vi "cont_array_float.vi"(7 "ignore_first_edge?":bool, 8 "edge cluster":cluster{"Array":i16[], "Array":bool[]}, 11 "u8_ar_phase map":dbl[](array[numeric])) -> (3 "Array":dbl[](array[numeric]))   [LabVIEW 2011]
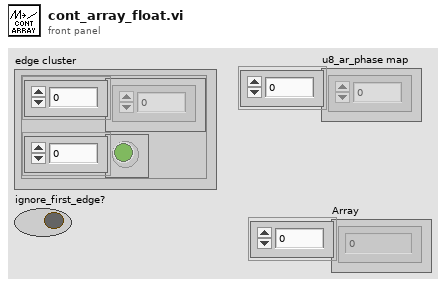
[diagram p1: front panel]
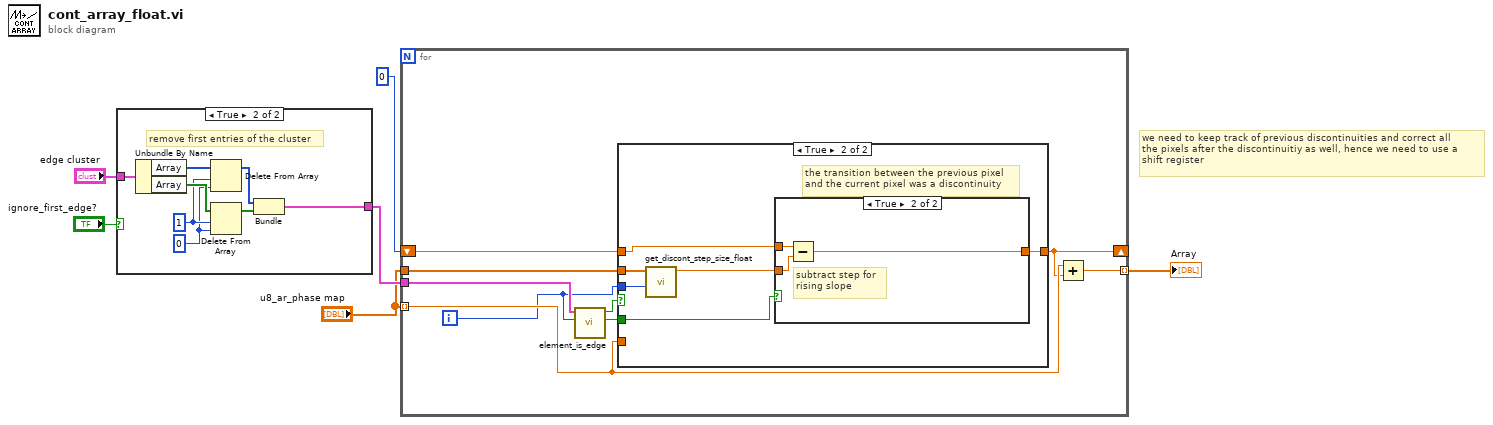
[diagram p0: block diagram]
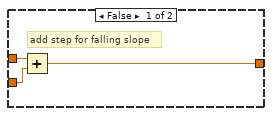
[diagram p4: hidden frame]
diagram:
  # "we need to keep track of previous discontinuities and correct all \nthe pixels after the discontinuitiy as well, hence we need to use a \nshift register"
  n1 = case shown="True" "ignore_first_edge?" {
    tunnel: "edge cluster" -> [w7 w9]
    tunnel: [w7 w8] -> w3
    frame False {
    }
    frame True {
      w13 = 1 ("length")
      w12 = 0 ("index")
      # "remove first entries of the cluster"
      n2 = Unbundle By Name(w9) -> ("Array"=w15:i16[], "Array"=w14:bool[])
      n3 = Delete From Array(array=w15, length=w13, index=w12) -> (array with subset deleted=w11:i16[])  [unwired: 1 out]
      n4 = Delete From Array(array=w14, length=w13, index=w12) -> (array with subset deleted=w10:bool[])  [unwired: 1 out]
      n5 = Bundle("Array"=w11, "Array"=w10) -> (w8:cluster{"Array":i16[], "Array":bool[]})  [unwired: 1 in]
    }
  }
  n6 = for {
    tunnel: "u8_ar_phase map" -> [w20]
    tunnel: "u8_ar_phase map" -> [w22] mode=indexing
    shift-right: [w19] -> _
    shift-left: i16 0 -> [w24]
    tunnel: [w23] -> w5 mode=indexing
    tunnel: w3 -> [w21]
    i -> [w18]
    n7 = call "element_is_edge.vi"("current element"=w18, "edge cluster"=w21) -> ("direction (rising/falling)"=w16:bool, "edge"=w17:bool)  [unwired: 8 in]
    n8 = case shown="True" w17 {
      tunnel: [w25 w30] -> w19
      tunnel: w24 -> [w25 w31]
      tunnel: w16 -> [_ w29]
      tunnel: w22 -> [_ _]
      tunnel: w18 -> [_ w27]
      tunnel: w20 -> [_ w28]
      frame False {
      }
      frame True {
        # "the transition between the previous pixel\nand the current pixel was a discontinuity"
        n9 = call "get_discont_step_size_float.vi"("current pixel (iteration)"=w27, "current row in image"=w28) -> ("step_size"=w26:dbl)  [unwired: 9 in]
        n10 = case shown="True" w29 {
          tunnel: w31 -> [w34 w37]
          tunnel: [w33 w36] -> w30
          tunnel: w26 -> [w32 w35]
          frame False {
            # "add step for falling slope"
            n11 = Add(x=w34, y=w32) -> (x+y=w33:dbl)
          }
          frame True {
            # "subtract step for \nrising slope"
            n12 = Subtract(x=w37, y=w35) -> (x-y=w36:dbl)
          }
        }
      }
    }
    n13 = Add(x=w22, y=w19) -> (x+y=w23:dbl)
  }
  "Array" <- w5
